vi "Write_Instr.vi"(8 "error in (no error)":errorcluster caption="entrée d'erreur (pas d'erreur)", 11 "Class Multimeter Power_Supply en entrée":refnum<class "Class Instrument Power_Supply.lvclass">) -> (0 "error out":errorcluster caption="sortie d'erreur", 3 "Class Multimeter Power_Supply en sortie":refnum<class "Class Instrument Power_Supply.lvclass">)   [LabVIEW 2020, in "Library Instrument & Equipement.lvlib" / "Library Instruments.lvlib" / "Class Instrument Power_Supply.lvclass"]
uses:
  Class Instrument Power_Supply.lvclass
  Class Instrument Power_Supply.lvclass/Class Instrument Power_Supply.ctl
  Instrument (Default)/Class Instrument (Default).lvclass
  Power_Supply/Power_Supply (Default)/Power_Supply (Default).lvclass
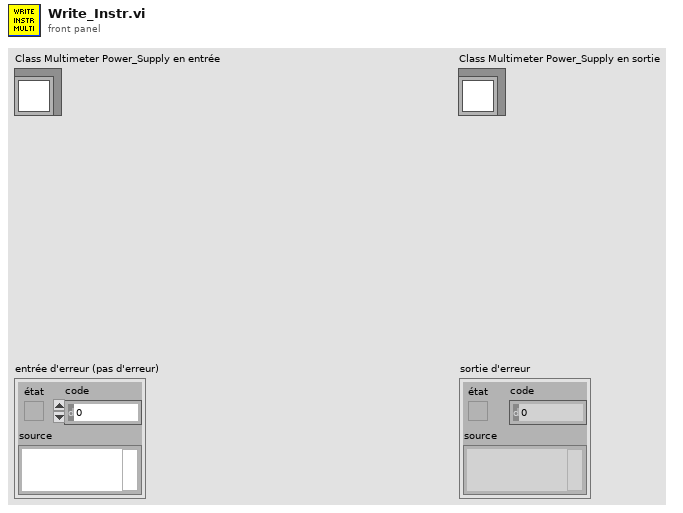
[diagram p1: front panel]
types:
  T1 = typedef "Library Commun.lvlib/Data_Write_Power_Supply.ctl" = enum16{"Enable Channel", "Disable Channel"}
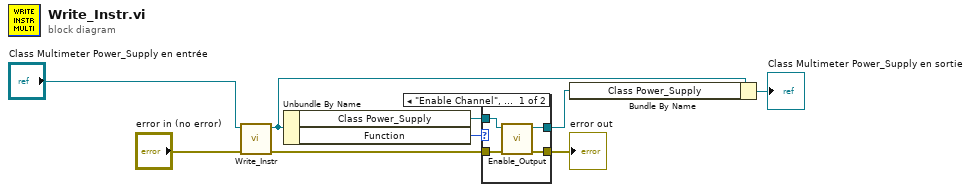
[diagram p0: block diagram]
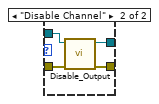
[diagram p2: hidden frame]
diagram:
  n1 = call-parent "Write_Instr.vi"("error in (no error)"="error in (no error)", "Class Multimeter (Default) en entrée"="Class Multimeter Power_Supply en entrée") -> ("error out"=w6:errorcluster, "Class Multimeter (Default) en sortie"=w2:refnum<class "Class Instrument Power_Supply.lvclass">)  [unwired: 8 in]
  n2 = Unbundle By Name(w2) -> ("Class Power_Supply"=w4:refnum<class "Power_Supply (Default).lvclass">, "Function"=w7:T1)
  n3 = case shown="\"Enable Channel\", Par défaut" w7 {
    tunnel: w6 -> [w12 w17]
    tunnel: [w11 w16] -> w5
    tunnel: w4 -> [w13 w15]
    tunnel: [w10 w14] -> w3
    frame "Enable Channel", Default {
      n4 = call-dynamic "Enable_Output.vi"("error in (no error)"=w12, "Power_Supply (Default) en entrée"=w13) -> ("error out"=w11:errorcluster, "Power_Supply (Default) en sortie"=w10:refnum<class "Power_Supply (Default).lvclass">)  [unwired: 8 in]
    }
    frame "Disable Channel" {
      n5 = call-dynamic "Disable_Output.vi"("error in (no error)"=w17, "Power_Supply (Default) en entrée"=w15) -> ("error out"=w16:errorcluster, "Power_Supply (Default) en sortie"=w14:refnum<class "Power_Supply (Default).lvclass">)  [unwired: 8 in]
    }
  }
  "error out" <- w5
  n6 = Bundle By Name(cluster=w2, "Class Power_Supply"=w3) -> (→"Class Multimeter Power_Supply en sortie":refnum<class "Class Instrument Power_Supply.lvclass">)
